vi "Monitoring PRF.vi"(6 "Measurement Type":enum32{"Volt", "SA"}(radio), 7 "error in (no error)":errorcluster, 9 "timeout (ms)":dbl=40000.0 format="%.2f", 10 "TCP from Orchid in":refnum<k5>) -> (0 "error out":errorcluster, 3 "PRF":dbl)   [LabVIEW 2016]
doc: "This VI sets the Z system transmit parameters for an intensity measurement, reads them back, and checks for errors. It first gets the initial center element delay (TxpgDelayAperA) and the system frequencies using tcpSysTxFreqFromZ.vi. It then sets the elevation aperture (using SetZElevAper.vi), channel modulation, wavestyle, frequency, focus, number of transmit elements, number of cycles, voltage, and voltage channel, in that order. It reads back the settings (using tcpReadIntenSettingsZ.vi) and checks for errors. The final trigger delay and change in delay, in microseconds, are calculated from the initial and final values of TxpgDelayAperA using:\ndelay(us) = (TxpgDelayAperA + 178.0) / 160"
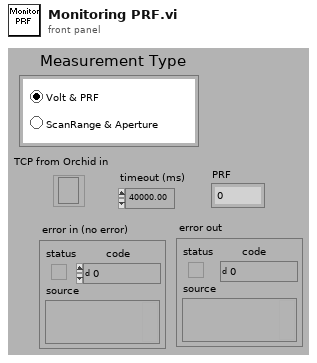
[diagram p1: front panel]
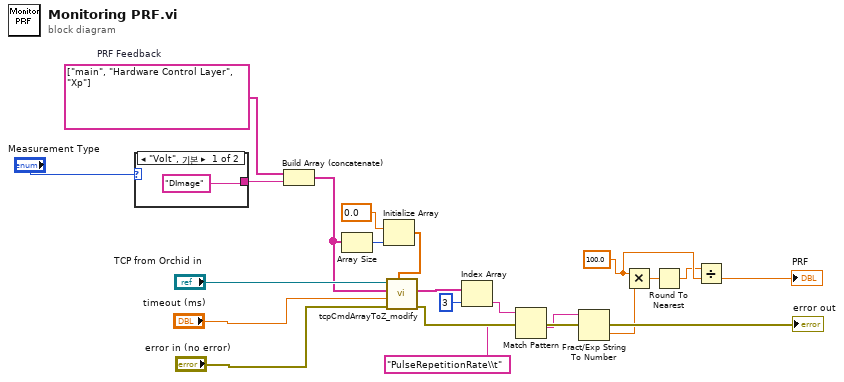
[diagram p0: block diagram]
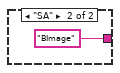
[diagram p2: hidden frame]
diagram:
  w3 = string[] ["main", "Hardware Control Layer", "Xp"]  # PRF Feedback
  w7 = 100.0
  n1 = case shown="\"Volt\", 기본" "Measurement Type" {
    tunnel: ["DImage" "BImage"] -> w2
    frame "Volt", Default {
    }
    frame "SA" {
    }
  }
  n2 = Build Array (concatenate)(w3, w2) -> (w1:string[])
  n3 = Array Size(array=w1) -> (size(s)=w14:i32)
  n4 = Initialize Array(0.0 ("element"), w14) -> (w16:dbl[])
  n5 = call "tcpCmdArrayToZ_modify.vi"("Delay (sec)"=w16, "error in (no error)"="error in (no error)", "Timeout (ms)"="timeout (ms)", "Command array"=w1, "connection ID in"="TCP from Orchid in") -> ("error out"=→"error out":errorcluster, "Receive array"=w13:string[])  [unwired: 2 in, 3 out]
  n6 = Index Array(array=w13, index=3) -> (element=w11:string)
  n7 = Match Pattern(string=w11, regular expression="PulseRepetitionRate\\t") -> (after substring=w9:string)  [unwired: 1 in, 3 out]
  n8 = Fract/Exp String To Number(string=w9) -> (number=w5:dbl)  [unwired: 3 in, 1 out]
  n9 = Multiply(x=w7, y=w5) -> (x*y=w8:dbl)
  n10 = Round To Nearest(number=w8) -> (nearest integer value=w6:dbl)
  n11 = Divide(x=w6, y=w7) -> (x/y=→"PRF":dbl)
